vi "G#Debugger_Highlight.vi"(1 "Tree":refnum<vi>, 2 "Aggregates":refnum<vi>, 3 "ObjectIDs":string[](array[string]), 5 "error in (no error)":errorcluster, 6 "AggregatesTags":refnum<vi>) -> (19 "error out":errorcluster)   [LabVIEW 2020, in "G#Debugger.lvlib"]
doc: "Highlights the specified objects in the tree view control."
uses:
  G#Debugger.lvlib
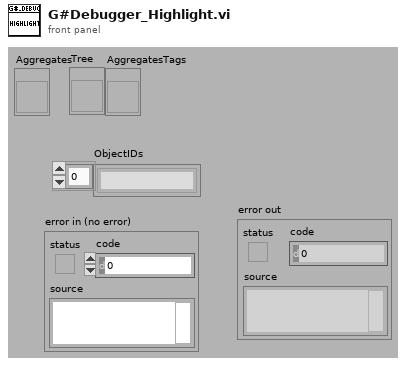
[diagram p1: front panel]
types:
  T1 = cluster{"Active Item Row Number":i32, "Class:Name":string, "object ID":string}
  T2 = cluster{"Active Item Row Number":i32, "Class:Name":string, "object ID":string}[]
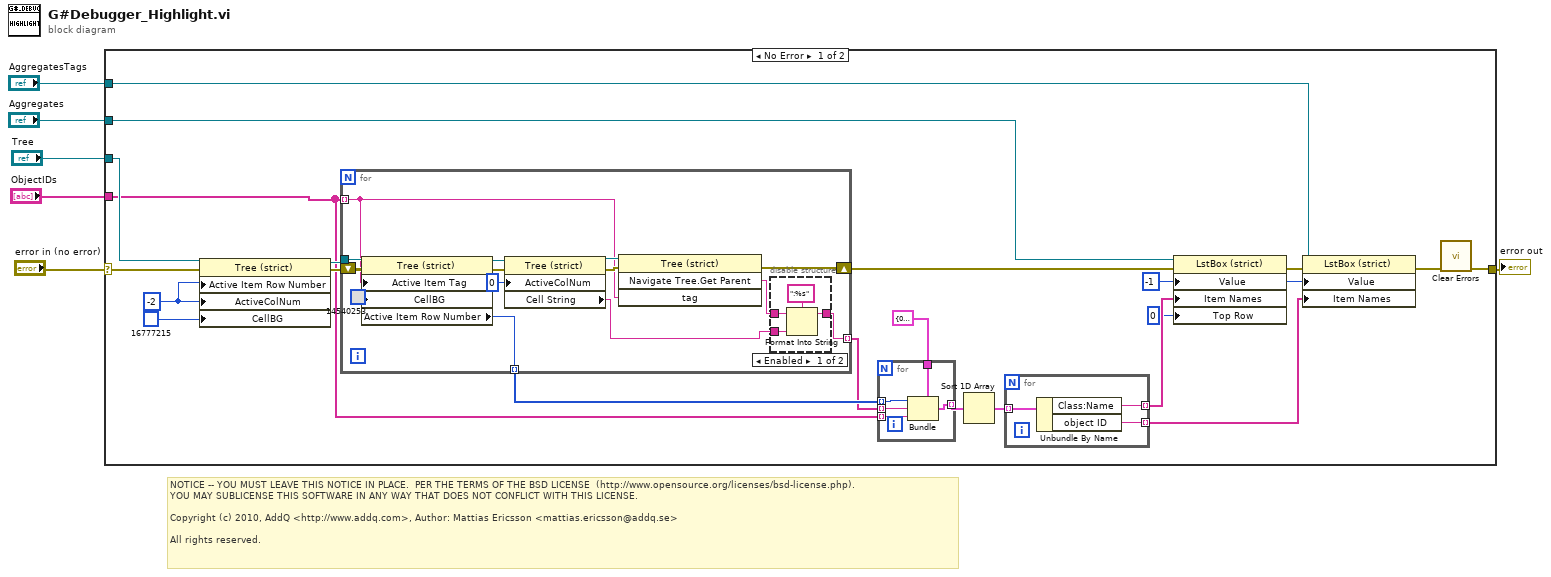
[diagram p0: block diagram]
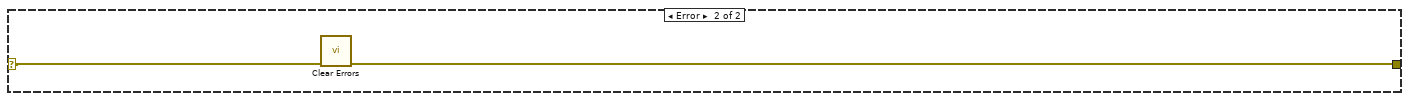
[diagram p3: hidden frame]
diagram:
  # "NOTICE -- YOU MUST LEAVE THIS NOTICE IN PLACE.  PER THE TERMS OF THE BSD LICENSE  (http://www.opensource.org/licenses/bsd-license.php).\nYOU MAY SUBLICENSE THIS SOFTWARE IN ANY WAY THAT DOES NOT CONFLICT WITH THIS LICENSE.\n\nCopyright (c) 2010, AddQ <http://www.addq.com>, Author: Mattias Ericsson <mattias.ericsson@addq.se>\n\nAll rights reserved."
  n1 = case shown="No Error" "error in (no error)" {
    selector: "error in (no error)" -> [w26 w57]
    tunnel: [w28 w56] -> w5
    tunnel: "Tree" -> [w24 _]
    tunnel: "ObjectIDs" -> [w9 _]
    tunnel: "Aggregates" -> [w21 _]
    tunnel: "AggregatesTags" -> [w16 _]
    frame No Error {
      w17 = -1 ("Value")
      w23 = -2 ("Active Cell:Active Column Number")
      n2 = property class="Tree (strict)"(reference=w24, error in=w26, "Active Item Row Number"=w23, "ActiveColNum"=w23, "CellBG"=u32 16777215 ("Color Box")) -> (reference out=w20:refnum<vi>, error out=w27:errorcluster)
      n3 = for {
        shift-right: [w42] -> w22
        shift-left: w27 -> [w49]
        tunnel: w9 -> [w41] mode=indexing
        tunnel: w20 -> [w50]
        tunnel: [w38] -> w12 mode=indexing
        tunnel: [w37] -> w15 mode=indexing
        n4 = property class="Tree (strict)"(reference=w50, error in=w49, "Active Item Tag"=w41, "CellBG"=u32 14540253 ("Color Box")) -> (reference out=w46:refnum<vi>, error out=w47:errorcluster, "Active Item Row Number"=w37:i32)
        n5 = property class="Tree (strict)"(reference=w46, error in=w47, "ActiveColNum"=0 ("Active Cell:Active Column Number")) -> (reference out=w44:refnum<vi>, error out=w43:errorcluster, "Cell String"=w39:string)
        n6 = invoke class="Tree (strict)" method="Navigate Tree.Get Parent"(reference=w44, error in=w43, "tag"=w41) -> (error out=w42:errorcluster, "Navigate Tree:Get Parent"=w40:string)  [unwired: 1 in, 2 out]
        n7 = disable-structure shown="Enabled" {
          disable-tunnel: w40 -> [w54 _]
          disable-tunnel: w39 -> [w52 w55]
          disable-tunnel: [w51 w55] -> w38
          frame Enabled {
            n8 = Format Into String(format string=":%s", initial string=w54, w52) -> (resulting string=w51:string)  [unwired: 1 in, 1 out]
          }
          frame Disabled {
          }
        }
      }
      n9 = for {
        tunnel: w15 -> [w35] mode=indexing
        tunnel: w12 -> [w36] mode=indexing
        tunnel: [w34] -> w14 mode=indexing
        tunnel: w9 -> [w33] mode=indexing
        tunnel: T1 {"Active Item Row Number"=0, "Class:Name"="", "object ID"=""} ("cluster") -> [w32]
        n10 = Bundle(cluster=w32, "Active Item Row Number"=w35, "Class:Name"=w36, "object ID"=w33) -> (w34:T1)
      }
      n11 = Sort 1D Array(array=w14) -> (sorted array=w13:T2)
      n12 = for {
        tunnel: w13 -> [w31] mode=indexing
        tunnel: [w30] -> w11 mode=indexing
        tunnel: [w29] -> w8 mode=indexing
        n13 = Unbundle By Name(w31) -> ("Class:Name"=w30:string, "object ID"=w29:string)
      }
      n14 = property on="Property Node" class="LstBox (strict)"(reference=w21, error in=w22, "Value"=w17, "Item Names"=w11, "Top Row"=0) -> (error out=w19:errorcluster)  [unwired: 1 out]
      n15 = property on="Property Node" class="LstBox (strict)"(reference=w16, error in=w19, "Value"=w17, "Item Names"=w8) -> (error out=w18:errorcluster)  [unwired: 1 out]
      n16 = call <vilib>:"Clear Errors.vi"("error in (no error)"=w18) -> ("error out"=w28:errorcluster)  [unwired: 5 in, 1 out]
    }
    frame Error {
      n17 = call <vilib>:"Clear Errors.vi"("error in (no error)"=w57) -> ("error out"=w56:errorcluster)  [unwired: 5 in, 1 out]
    }
  }
  "error out" <- w5
